vi "Build Fail Message.vi"(8 "Test Name":string, 9 "Lower Limit":refnum<class "Const_DBL.lvclass">, 10 "Upper Limit":refnum<class "Const_DBL.lvclass">, 11 "Result":refnum<class "Abs_Double Float.lvclass">) -> (3 "Abs_String out":refnum<class "Abs_String.lvclass">)   [LabVIEW 2021, in "Test Sequencer Support.lvlib"]
uses:
  <vilib>/TSA/Abstract Data Classes/Constants/Support/DBL/Const_DBL.lvclass
  C:/Program Files (x86)/National Instruments/LabVIEW 2021/vi.lib/TSA/Abstract Data Classes/Abs_Types/Value/Abs_Value.lvclass
  <vilib>/TSA/Abstract Data Classes/Abs_Types/Double Float/Abs_Double Float.lvclass
  <vilib>/TSA/Abstract Data Classes/Abs_Types/String/Abs_String.lvclass
  <vilib>/TSA/Abstract Data Classes/Constants/Support/Str/Str.vi
  Test Sequencer Support.lvlib
  <vilib>/TSA/Abstract Data Classes/Constants/Support/Str/Const_Str.lvclass
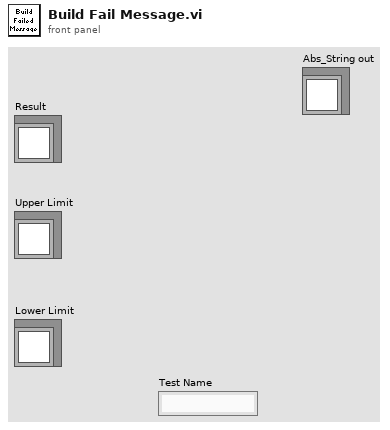
[diagram p1: front panel]
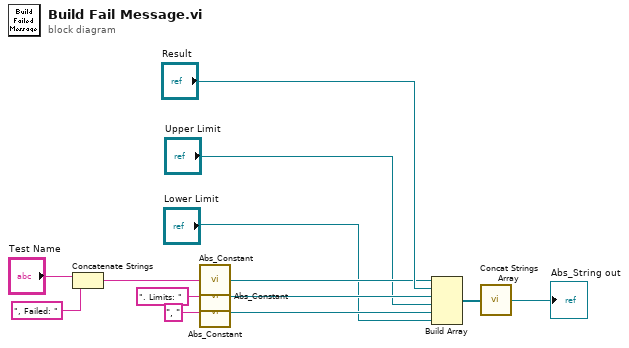
[diagram p0: block diagram]
diagram:
  n1 = Concatenate Strings("Test Name", ", Failed: " ("string")) -> (w4:string)
  n2 = call-poly <vilib>:"Abs_Constant.vi"("String"=w4) -> ("Abs_String.lvclass"=w8:refnum<class "Abs_String.lvclass">)  [unwired: 4 in]
  n3 = call-poly <vilib>:"Abs_Constant.vi"("String"=". Limits: " ("Name")) -> ("Abs_String.lvclass"=w11:refnum<class "Abs_String.lvclass">)  [unwired: 4 in]
  n4 = call-poly <vilib>:"Abs_Constant.vi"("String"=", " ("Name")) -> ("Abs_String.lvclass"=w13:refnum<class "Abs_String.lvclass">)  [unwired: 4 in]
  n5 = Build Array(w8, "Result", w11, "Upper Limit", w13, "Lower Limit") -> (w5:refnum<class "Abs_Value.lvclass">[])
  n6 = call <vilib>:"Concat Strings Array.vi"("Strings"=w5) -> ("Result"=→"Abs_String out":refnum<class "Abs_String.lvclass">)  [unwired: 4 in]
